vi "Calculate_Timescales_exp.vi"(1 "Sampling Frequency (Hz)":dbl, 2 "Autocorrelation length":i32, 3 "Autocorrelation":dbl[](array[numeric])) -> (0 "Time Scale estimate (s)":dbl)   [LabVIEW 2011]
uses:
  <vilib>/Analysis/NI_AALPro.lvlib
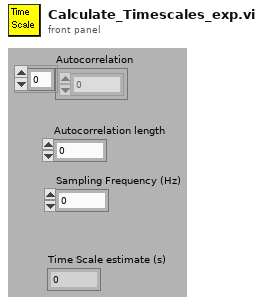
[diagram p1: front panel]
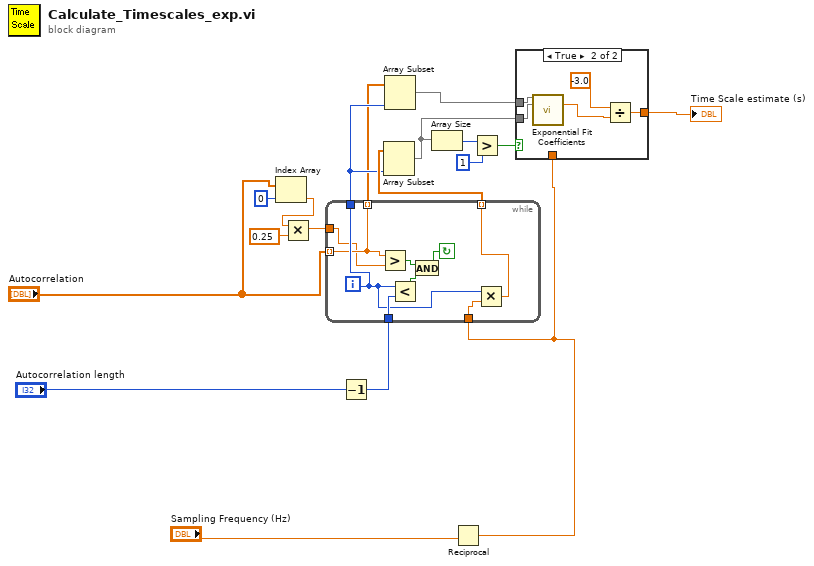
[diagram p0: block diagram]
diagram:
  n1 = Index Array(array="Autocorrelation", index=0) -> (element=w16:dbl)
  n2 = Multiply(x=w16, y=0.25) -> (x*y=w18:dbl)
  n3 = Decrement(x="Autocorrelation length") -> (x-1=w1:i32)
  n4 = Reciprocal(x="Sampling Frequency (Hz)") -> (1/x=w3:dbl)
  n5 = while {
    tunnel: "Autocorrelation" -> [w21] mode=indexing
    tunnel: w1 -> [w27]
    tunnel: w3 -> [w24]
    tunnel: [w23] -> w7 mode=indexing
    tunnel: [w21] -> w5 mode=indexing
    tunnel: [w22] -> w6
    tunnel: w18 -> [w20]
    i -> [w22]
    stop <- w25 continue-if-true
    n6 = Greater?(x=w21, y=w20) -> (0:w19:bool)
    n7 = Less?(x=w22, y=w27) -> (x < y?=w26:bool)
    n8 = And(x=w19, y=w26) -> (x .and. y?=w25:bool)
    n9 = Multiply(x=w22, y=w24) -> (x*y=w23:dbl)
  }
  n10 = Array Subset(array=w7, length=w6) -> (w12:dbl[])  [unwired: 1 in]
  n11 = Array Subset(array=w5, length=w6) -> (w11:dbl[])  [unwired: 1 in]
  n12 = Array Size(array=w12) -> (size(s)=w9:i32)
  n13 = Greater?(x=w9, y=1) -> (0:w13:bool)
  n14 = case shown="True" w13 {
    tunnel: [w28 w32] -> w8
    tunnel: w11 -> [_ w31]
    tunnel: w12 -> [_ w29]
    tunnel: w3 -> [w28 _]
    frame False {
    }
    frame True {
      n15 = call <vilib>:"Exponential Fit Coefficients.vi"("Y"=w31, "X"=w29) -> ("damping"=w30:dbl)  [unwired: 11 in, 2 out]
      n16 = Divide(x=-3.0, y=w30) -> (x/y=w32:dbl)
    }
  }
  "Time Scale estimate (s)" <- w8
